vi "transport char run.vi"() -> ()   [LabVIEW 2009]
uses:
  <vilib>/Utility/file.llb/Write To Spreadsheet File (DBL).vi
panel:
  in  "MAXIMUM":ext format="%.2e"
  in  "MINIMUM":ext=-1e-05 format="%_2e"
  out "graphic display 2":cluster{"trace":dbl[], "trace":dbl[]}(graph)
  in  "Y1 axis":string="Id"
  in  "Y2 axis settings":T1={"Y2 axis on/off"=FALSE, "MINIMUM"=-1e-07, "MAXIMUM"=1e-07, "Variable name"="", "LIN or LOG axis"=""} {"MAXIMUM" format="%.2e"; "MINIMUM" format="%.2e"}
  in  "VISA session":refnum<visa-resource-name>="GPIB0::17::INSTR"
  out "graphic display":cluster{"trace":dbl[], "trace":dbl[]}(graph)
  in  "Var2 step settings":T2={"compliance (A)"=0.001, "compliance (V)"=100.0, "start"=0.0, "total points"=7, "step"=-10.0} {"step" format="%.2f"; "start" format="%.2f"; "compliance (V)" format="%.2f"; "compliance (A)" format="%^.2e"}
  in  "wait time parameter":dbl=1.0
  in  "integration time":u32(slide) scale=0.0..2.0
  in  "Var1 sweep settings":T3={"start"=0.0, "stop"=-60.0, "step (linear only)"=-1.0, "sweep spacing (linear: 0)"=0, "sweep mode"=FALSE, "compliance (V)"=100.0, "compliance (A)"=0.001} {"compliance (A)" format="%^.2e"; "compliance (V)" format="%.2f"; "sweep spacing (linear: 0)" items=["linear", "log 10", "log 25", "log 50"]; "step (linear only)" format="%.2f"; "stop" format="%.2f"; "start" format="%.2f"}
  in  "Value (Either V or A) 4":dbl
  in  "Value (Either V or A) 3":dbl
  in  "Value (Either V or A) 2":dbl
  in  "Value (V or A)":dbl
  in  "compliance (A)":dbl=0.001 format="%^.2e"
  in  "compliance (V)":dbl=100.0 format="%^.2e"
  out "error?":errorcluster
  in  "Iname":string="Is"
  in  "Vname":string="Vs"
  in  "Function":u16(ring)=4 items=["disabled", "Var1", "Var2", "Var1'", "Constant"]
  in  "Mode":u16(ring)=4 items=["V", "I", "VPulse", "IPulse", "Common"]
  in  "Iname 4":string="I4"
  in  "Vname 4":string="V4"
  in  "Function 4":u16(ring)=4 items=["disabled", "Var1", "Var2", "Var1'", "Constant"]
  in  "Mode 4":u16(ring) items=["V", "I", "VPulse", "IPulse", "Common"]
  in  "Iname 3":string="Ig"
  in  "Vname 3":string="Vg"
  in  "Function 3":u16(ring)=2 items=["disabled", "Var1", "Var2", "Var1'", "Constant"]
  in  "Mode 3":u16(ring) items=["V", "I", "VPulse", "IPulse", "Common"]
  in  "Iname 2":string="Id"
  in  "Vname 2":string="Vd"
  in  "Function 2":u16(ring)=1 items=["disabled", "Var1", "Var2", "Var1'", "Constant"]
  in  "Mode 2":u16(ring) items=["V", "I", "VPulse", "IPulse", "Common"]
  in  "reset":bool=TRUE
  # "SMU1"
  # "SMU2"
  # "SMU3"
  # "SMU4"
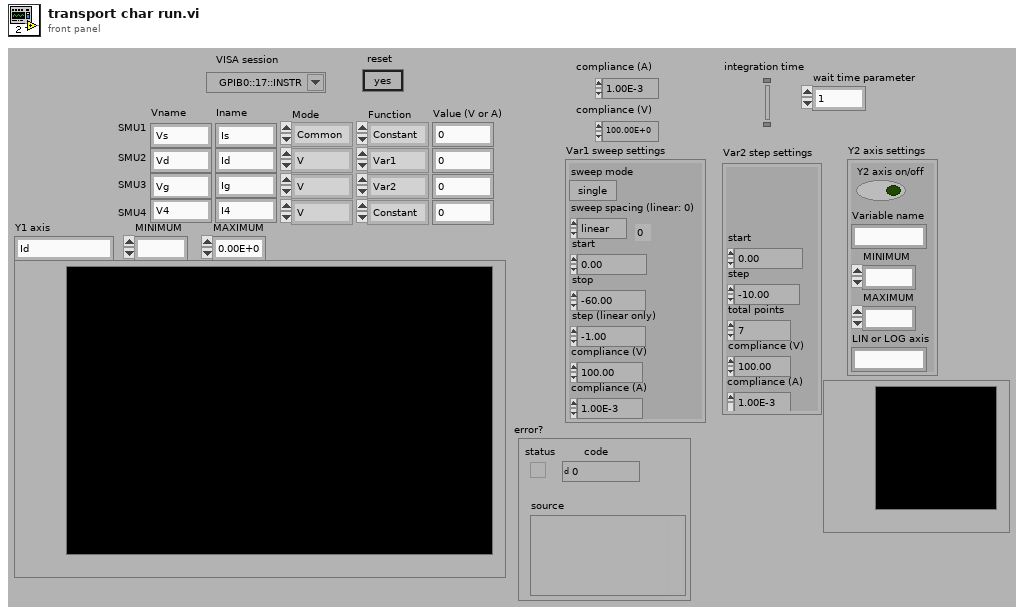
[diagram p1: front panel]
types:
  T1 = cluster{"Y2 axis on/off":bool, "MINIMUM":ext, "MAXIMUM":ext, "Variable name":string, "LIN or LOG axis":string}
  T2 = cluster{"compliance (A)":dbl, "compliance (V)":dbl, "start":dbl, "total points":u16, "step":dbl}
  T3 = cluster{"start":dbl, "stop":dbl, "step (linear only)":dbl, "sweep spacing (linear: 0)":u16, "sweep mode":bool, "compliance (V)":dbl, "compliance (A)":dbl}
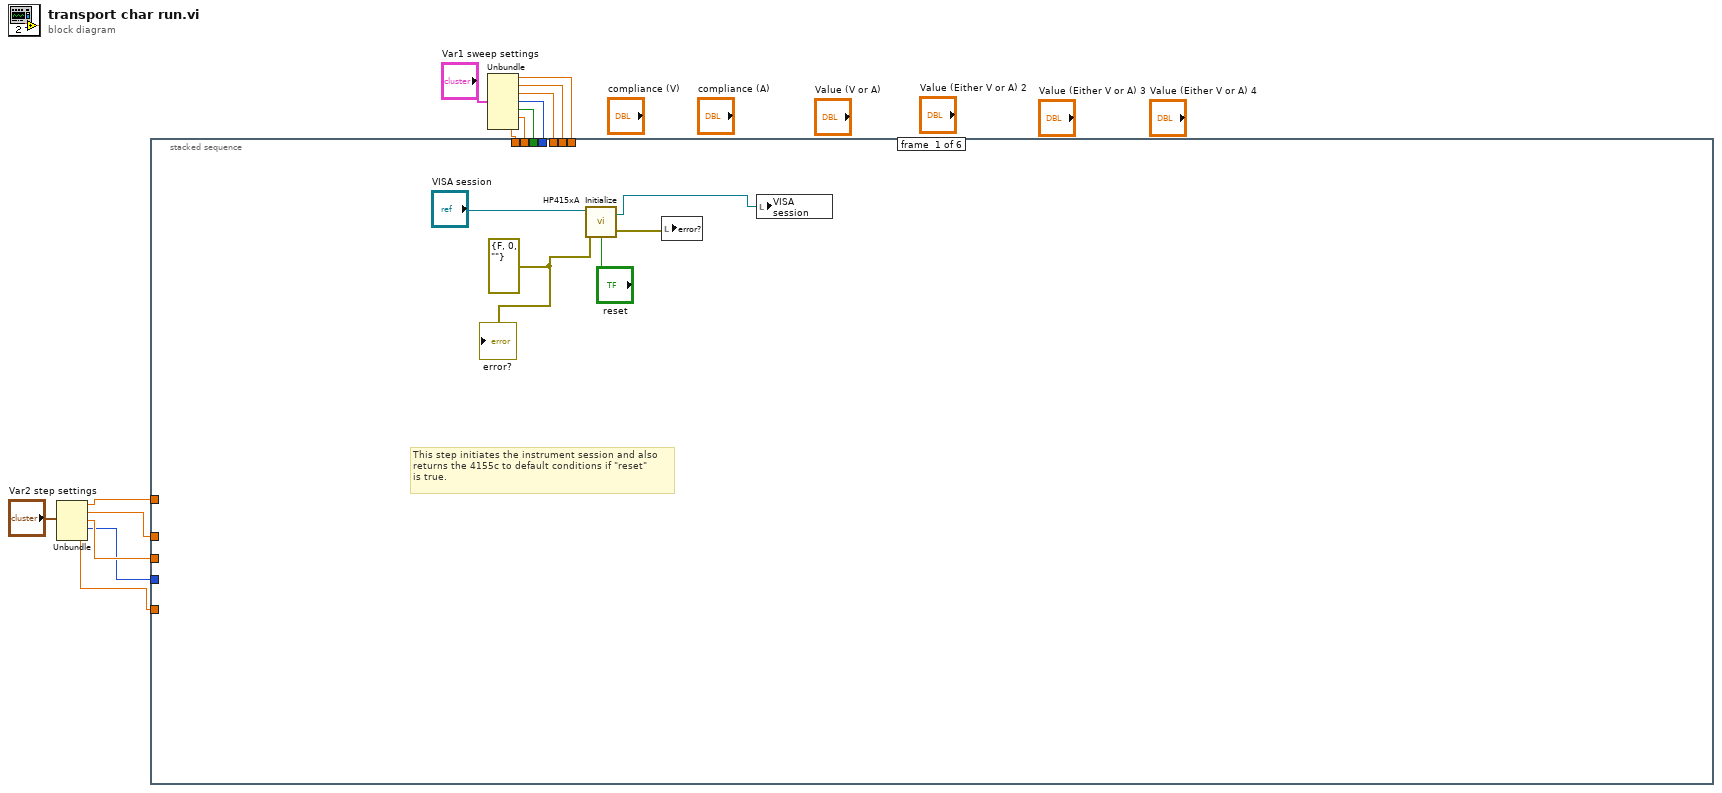
[diagram p0: block diagram]
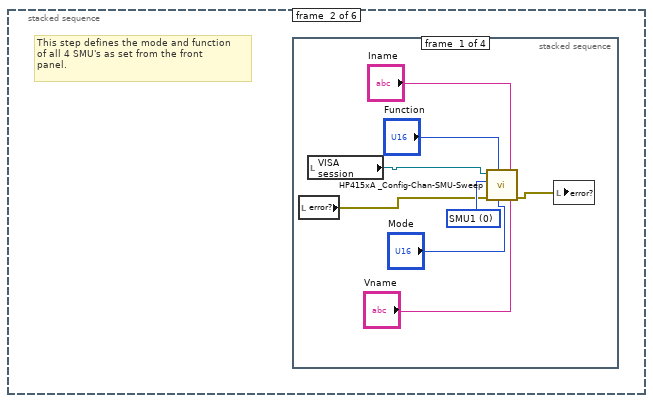
[diagram p2: hidden frame]
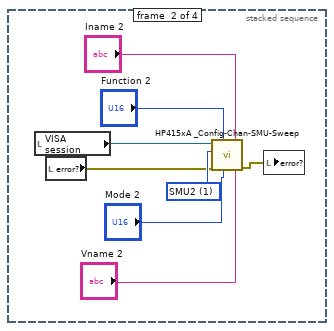
[diagram p3: hidden frame]
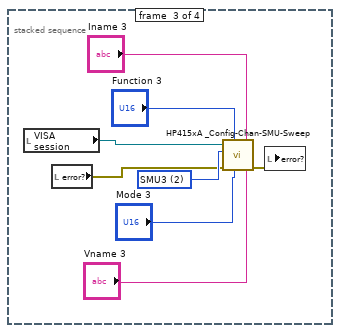
[diagram p4: hidden frame]
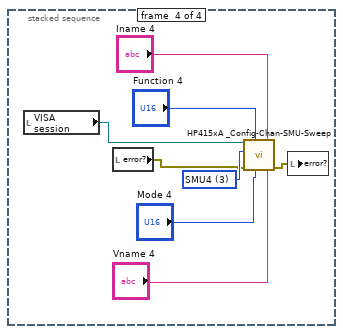
[diagram p5: hidden frame]
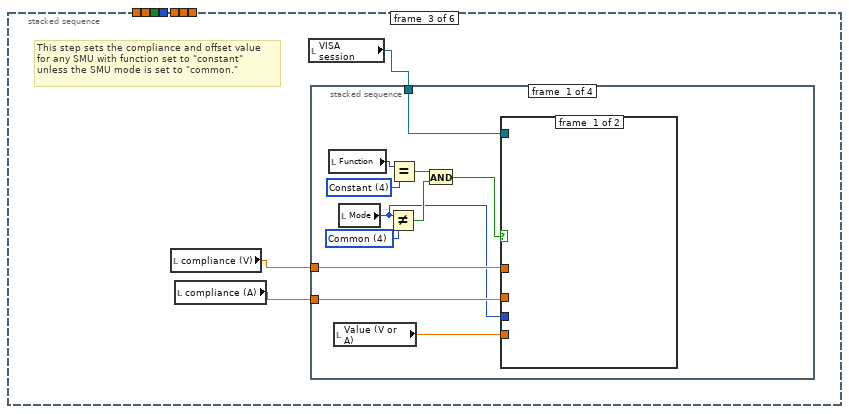
[diagram p6: hidden frame]
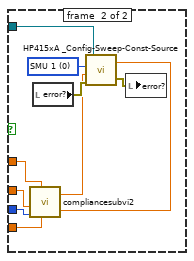
[diagram p7: hidden frame]
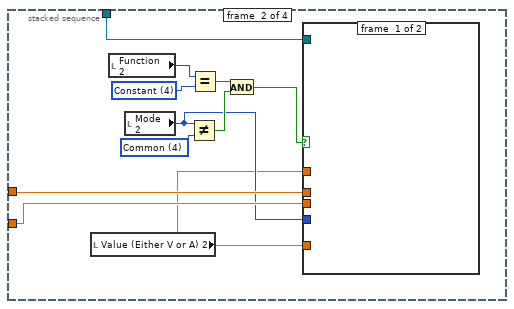
[diagram p8: hidden frame]
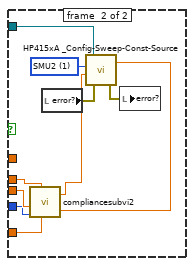
[diagram p9: hidden frame]
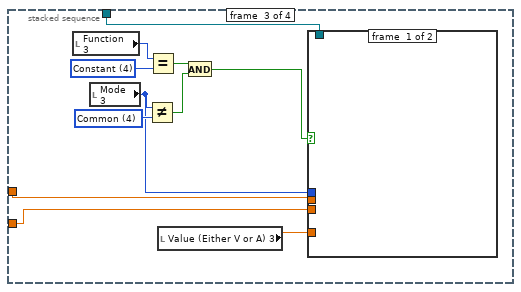
[diagram p10: hidden frame]
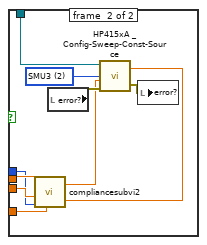
[diagram p11: hidden frame]
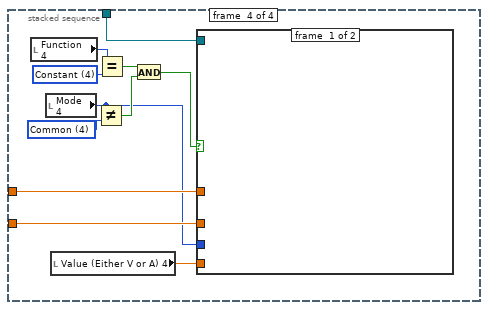
[diagram p12: hidden frame]
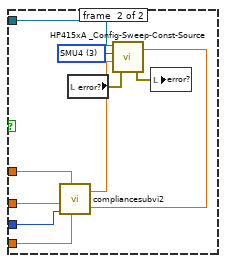
[diagram p13: hidden frame]
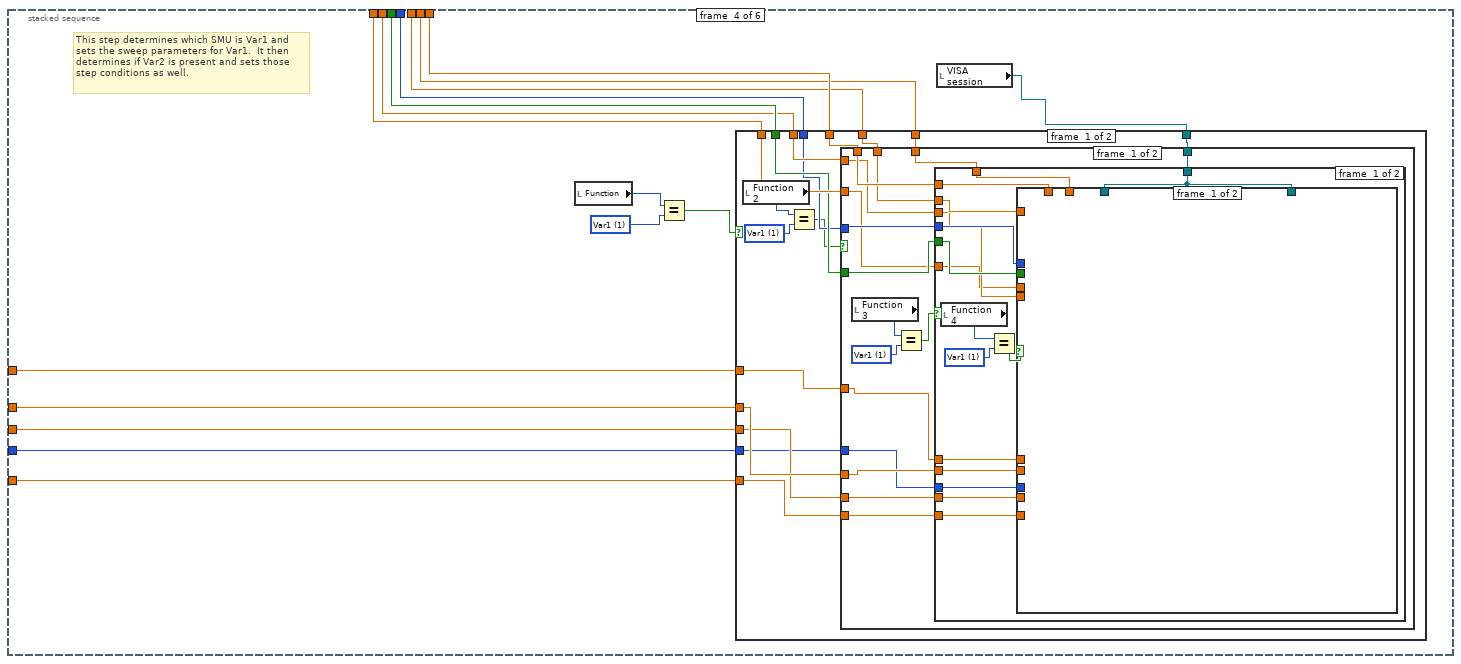
[diagram p14: hidden frame]
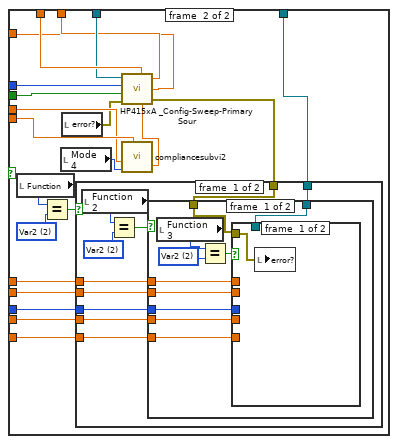
[diagram p15: hidden frame]
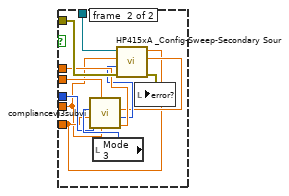
[diagram p16: hidden frame]
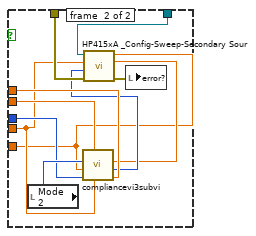
[diagram p17: hidden frame]
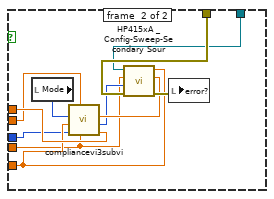
[diagram p18: hidden frame]
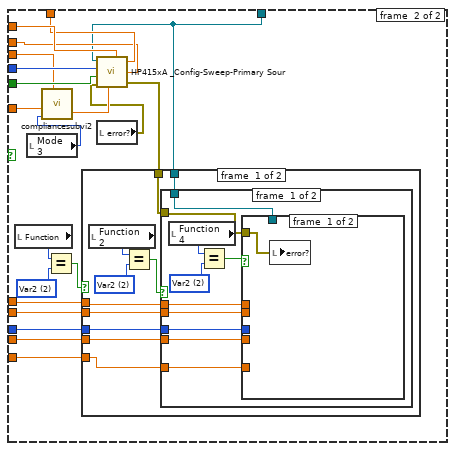
[diagram p19: hidden frame]
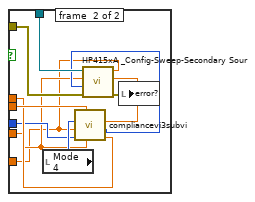
[diagram p20: hidden frame]
diagram:
  n1 = Unbundle("Var2 step settings") -> ("compliance (A)"=w5:dbl, "compliance (V)"=w4:dbl, "start"=w3:dbl, "total points"=w2:u16, "step"=w1:dbl)
  n2 = Unbundle("Var1 sweep settings") -> ("start"=w13:dbl, "stop"=w12:dbl, "step (linear only)"=w11:dbl, "sweep spacing (linear: 0)"=w10:u16, "sweep mode"=w9:bool, "compliance (V)"=w8:dbl, "compliance (A)"=w7:dbl)
  n3 = stacked-sequence {
    tunnel: w13 -> [_ _ _ w150 _ _]
    tunnel: w12 -> [_ _ _ w149 _ _]
    tunnel: w11 -> [_ _ _ w148 _ _]
    tunnel: w10 -> [_ _ _ w147 _ _]
    tunnel: w9 -> [_ _ _ w146 _ _]
    tunnel: w8 -> [_ _ _ w145 _ _]
    tunnel: w7 -> [_ _ _ w144 _ _]
    tunnel: w5 -> [_ _ _ w143 _ _]
    tunnel: w4 -> [_ _ _ w142 _ _]
    tunnel: w3 -> [_ _ _ w141 _ _]
    tunnel: w2 -> [_ _ _ w140 _ _]
    tunnel: w1 -> [_ _ _ w139 _ _]
    frame #0 {
      w18 = errorcluster {"status"=FALSE, "code"=0, "source"=""} ("error out")
      # "This step initiates the instrument session and also\nreturns the 4155c to default conditions if \"reset\"\nis true."
      n4 = call "HP415xA  Initialize.vi"("instrument descriptor"="VISA session", "reset"="reset", "error in (no error)"=w18) -> ("VISA session"=w15:refnum<visa-resource-name>, "error out"=w17:errorcluster)  [unwired: 2 in]
      n5 = local write "error?"(w17) -> ()
      n6 = local write "VISA session"(w15) -> ()
      "error?" <- w18
    }
    frame #1 {
      # "This step defines the mode and function\nof all 4 SMU's as set from the front\npanel."
      n7 = stacked-sequence {
        frame #0 {
          w27 = u32 0 items=["SMU1  ", "SMU2  ", "SMU3  ", "SMU4  ", "SMU5  ", "SMU6  "] ("unit to configure")
          n8 = local read "error?"() -> (w22:errorcluster)
          n9 = local read "VISA session"() -> (w20:refnum<visa-resource-name>)
          n10 = call "HP415xA _Config-Chan-SMU-Sweep.vi"("V name (max 6 chars)"="Vname", "I name (max 6 chars)"="Iname", "mode"="Mode", "function"="Function", "error in (no error)"=w22, "unit to configure"=w27, "VISA session"=w20) -> ("error out"=w21:errorcluster)  [unwired: 2 in]
          n11 = local write "error?"(w21) -> ()
        }
        frame #1 {
          w31 = u32 1 items=["SMU1  ", "SMU2  ", "SMU3  ", "SMU4  ", "SMU5  ", "SMU6  "] ("unit to configure")
          n12 = local read "VISA session"() -> (w28:refnum<visa-resource-name>)
          n13 = local read "error?"() -> (w29:errorcluster)
          n14 = call "HP415xA _Config-Chan-SMU-Sweep.vi"("V name (max 6 chars)"="Vname 2", "I name (max 6 chars)"="Iname 2", "mode"="Mode 2", "function"="Function 2", "error in (no error)"=w29, "unit to configure"=w31, "VISA session"=w28) -> ("error out"=w30:errorcluster)  [unwired: 2 in]
          n15 = local write "error?"(w30) -> ()
        }
        frame #2 {
          w39 = u32 2 items=["SMU1  ", "SMU2  ", "SMU3  ", "SMU4  ", "SMU5  ", "SMU6  "] ("unit to configure")
          n16 = local read "VISA session"() -> (w36:refnum<visa-resource-name>)
          n17 = local read "error?"() -> (w37:errorcluster)
          n18 = call "HP415xA _Config-Chan-SMU-Sweep.vi"("V name (max 6 chars)"="Vname 3", "I name (max 6 chars)"="Iname 3", "mode"="Mode 3", "function"="Function 3", "error in (no error)"=w37, "unit to configure"=w39, "VISA session"=w36) -> ("error out"=w38:errorcluster)  [unwired: 2 in]
          n19 = local write "error?"(w38) -> ()
        }
        frame #3 {
          w47 = u32 3 items=["SMU1  ", "SMU2  ", "SMU3  ", "SMU4  ", "SMU5  ", "SMU6  "] ("unit to configure")
          n20 = local read "VISA session"() -> (w44:refnum<visa-resource-name>)
          n21 = local read "error?"() -> (w46:errorcluster)
          n22 = call "HP415xA _Config-Chan-SMU-Sweep.vi"("V name (max 6 chars)"="Vname 4", "I name (max 6 chars)"="Iname 4", "mode"="Mode 4", "function"="Function 4", "error in (no error)"=w46, "unit to configure"=w47, "VISA session"=w44) -> ("error out"=w45:errorcluster)  [unwired: 2 in]
          n23 = local write "error?"(w45) -> ()
        }
      }
    }
    frame #2 {
      # "This step sets the compliance and offset value\nfor any SMU with function set to \"constant\"\nunless the SMU mode is set to \"common.\""
      n24 = local read "compliance (V)"() -> (w53:dbl)
      n25 = local read "compliance (A)"() -> (w54:dbl)
      n26 = local read "VISA session"() -> (w52:refnum<visa-resource-name>)
      n27 = stacked-sequence {
        tunnel: w52 -> [w63 w83 w102 w122]
        tunnel: w54 -> [w57 w79 w100 w120]
        tunnel: w53 -> [w56 w78 w99 w121]
        frame #0 {
          w61 = u16 4 items=["V", "I", "VPulse", "IPulse", "Common"] ("Mode")
          w65 = u16 4 items=["disabled", "Var1", "Var2", "Var1'", "Constant"] ("Function")
          n28 = local read "Function"() -> (w64:u16)
          n29 = local read "Value (V or A)"() -> (w58:dbl)
          n30 = local read "Mode"() -> (w55:u16)
          n31 = Not Equal?(x=w55, y=w61) -> (x != y?=w60:bool)
          n32 = Equal?(x=w64, y=w65) -> (x = y?=w62:bool)
          n33 = And(x=w62, y=w60) -> (x .and. y?=w59:bool)
          n34 = case shown="False" w59 {
            tunnel: w63 -> [_ w75]
            tunnel: w56 -> [_ w71]
            tunnel: w57 -> [_ w70]
            tunnel: w58 -> [_ w67]
            tunnel: w55 -> [_ w68]
            frame #0 {
            }
            frame #1 {
              w74 = u16 0 items=["SMU 1", "SMU2", "SMU3", "SMU4", "SMU5", "SMU6", "VSU1", "VSU2"] ("unit (SMU1:0)")
              n35 = call "compliancesubvi2.vi"("Value1"=w67, "compliance (V)"=w71, "Mode"=w68, "compliance (A)"=w70) -> ("compliance"=w69:dbl, "constant"=w66:dbl)  [unwired: 2 in]
              n36 = local read "error?"() -> (w73:errorcluster)
              n37 = call "HP415xA _Config-Sweep-Const-Source.vi"("compliance (SMUs only)"=w69, "error in (no error)"=w73, "source (V or A)"=w66, "unit (SMU1:0)"=w74, "VISA session"=w75) -> ("error out"=w72:errorcluster)
              n38 = local write "error?"(w72) -> ()
            }
          }
        }
        frame #1 {
          w80 = u16 4 items=["V", "I", "VPulse", "IPulse", "Common"] ("Mode 2")
          w81 = u16 4 items=["disabled", "Var1", "Var2", "Var1'", "Constant"] ("Function 2")
          n39 = local read "Value (Either V or A) 2"() -> (w76:dbl)
          n40 = local read "Function 2"() -> (w82:u16)
          n41 = local read "Mode 2"() -> (w77:u16)
          n42 = Not Equal?(x=w77, y=w80) -> (x != y?=w85:bool)
          n43 = Equal?(x=w82, y=w81) -> (x = y?=w86:bool)
          n44 = And(x=w86, y=w85) -> (x .and. y?=w84:bool)
          n45 = case shown="False" w84 {
            tunnel: w83 -> [_ w96]
            tunnel: w78 -> [_ w94]
            tunnel: w79 -> [_ w93]
            tunnel: w76 -> [_ _]
            tunnel: w77 -> [_ w89]
            tunnel: w76 -> [_ w88]
            frame #0 {
            }
            frame #1 {
              w95 = u16 1 items=["SMU 1", "SMU2", "SMU3", "SMU4", "SMU5", "SMU6", "VSU1", "VSU2"] ("unit (SMU1:0)")
              n46 = call "compliancesubvi2.vi"("Value1"=w88, "compliance (V)"=w94, "Mode"=w89, "compliance (A)"=w93) -> ("compliance"=w92:dbl, "constant"=w87:dbl)  [unwired: 2 in]
              n47 = local read "error?"() -> (w91:errorcluster)
              n48 = call "HP415xA _Config-Sweep-Const-Source.vi"("compliance (SMUs only)"=w92, "error in (no error)"=w91, "source (V or A)"=w87, "unit (SMU1:0)"=w95, "VISA session"=w96) -> ("error out"=w90:errorcluster)
              n49 = local write "error?"(w90) -> ()
            }
          }
        }
        frame #2 {
          w104 = u16 4 items=["V", "I", "VPulse", "IPulse", "Common"] ("Mode 2")
          w105 = u16 4 items=["disabled", "Var1", "Var2", "Var1'", "Constant"] ("Function 2")
          n50 = local read "Function 3"() -> (w103:u16)
          n51 = local read "Mode 3"() -> (w98:u16)
          n52 = Not Equal?(x=w98, y=w104) -> (x != y?=w106:bool)
          n53 = Equal?(x=w103, y=w105) -> (x = y?=w107:bool)
          n54 = local read "Value (Either V or A) 3"() -> (w101:dbl)
          n55 = And(x=w107, y=w106) -> (x .and. y?=w97:bool)
          n56 = case shown="False" w97 {
            tunnel: w102 -> [_ w115]
            tunnel: w101 -> [_ w109]
            tunnel: w100 -> [_ w112]
            tunnel: w99 -> [_ w111]
            tunnel: w98 -> [_ w110]
            frame #0 {
            }
            frame #1 {
              w114 = u16 2 items=["SMU 1", "SMU2", "SMU3", "SMU4", "SMU5", "SMU6", "VSU1", "VSU2"] ("unit (SMU1:0)")
              n57 = call "compliancesubvi2.vi"("Value1"=w109, "compliance (V)"=w111, "Mode"=w110, "compliance (A)"=w112) -> ("compliance"=w113:dbl, "constant"=w108:dbl)  [unwired: 2 in]
              n58 = local read "error?"() -> (w117:errorcluster)
              n59 = call "HP415xA _Config-Sweep-Const-Source.vi"("compliance (SMUs only)"=w113, "error in (no error)"=w117, "source (V or A)"=w108, "unit (SMU1:0)"=w114, "VISA session"=w115) -> ("error out"=w116:errorcluster)
              n60 = local write "error?"(w116) -> ()
            }
          }
        }
        frame #3 {
          w124 = u16 4 items=["V", "I", "VPulse", "IPulse", "Common"] ("Mode 4")
          w125 = u16 4 items=["disabled", "Var1", "Var2", "Var1'", "Constant"] ("Function 4")
          n61 = local read "Function 4"() -> (w126:u16)
          n62 = local read "Mode 4"() -> (w119:u16)
          n63 = local read "Value (Either V or A) 4"() -> (w118:dbl)
          n64 = Not Equal?(x=w119, y=w124) -> (x != y?=w127:bool)
          n65 = Equal?(x=w126, y=w125) -> (x = y?=w128:bool)
          n66 = And(x=w128, y=w127) -> (x .and. y?=w123:bool)
          n67 = case shown="True" w123 {
            tunnel: w122 -> [_ w137]
            tunnel: w121 -> [_ w133]
            tunnel: w120 -> [_ w134]
            tunnel: w119 -> [_ w132]
            tunnel: w118 -> [_ w131]
            frame #0 {
            }
            frame #1 {
              w138 = u16 3 items=["SMU 1", "SMU2", "SMU3", "SMU4", "SMU5", "SMU6", "VSU1", "VSU2"] ("unit (SMU1:0)")
              n68 = call "compliancesubvi2.vi"("Value1"=w131, "compliance (V)"=w133, "Mode"=w132, "compliance (A)"=w134) -> ("compliance"=w130:dbl, "constant"=w129:dbl)  [unwired: 2 in]
              n69 = local read "error?"() -> (w136:errorcluster)
              n70 = call "HP415xA _Config-Sweep-Const-Source.vi"("compliance (SMUs only)"=w130, "error in (no error)"=w136, "source (V or A)"=w129, "unit (SMU1:0)"=w138, "VISA session"=w137) -> ("error out"=w135:errorcluster)
              n71 = local write "error?"(w135) -> ()
            }
          }
        }
      }
    }
    frame #3 {
      w154 = u16 1 items=["disabled", "Var1", "Var2", "Var1'", "Constant"] ("Function")
      # "This step determines which SMU is Var1 and\nsets the sweep parameters for Var1.  It then\ndetermines if Var2 is present and sets those\nstep conditions as well."
      n72 = local read "Function"() -> (w153:u16)
      n73 = Equal?(x=w153, y=w154) -> (x = y?=w152:bool)
      n74 = local read "VISA session"() -> (w151:refnum<visa-resource-name>)
      n75 = case shown="False" w152 {
        tunnel: w145 -> [w167 w443]
        tunnel: w144 -> [w168 w442]
        tunnel: w147 -> [w165 w441]
        tunnel: w146 -> [w166 w440]
        tunnel: w148 -> [w162 w439]
        tunnel: w149 -> [w161 w438]
        tunnel: w150 -> [w163 w437]
        tunnel: w151 -> [w164 w426]
        tunnel: w143 -> [w159 w432]
        tunnel: w142 -> [w158 w431]
        tunnel: w141 -> [w157 w430]
        tunnel: w140 -> [w156 w429]
        tunnel: w139 -> [w155 w428]
        frame #0 {
          w170 = u16 1 items=["disabled", "Var1", "Var2", "Var1'", "Constant"] ("Function")
          n76 = local read "Function 2"() -> (w169:u16)
          n77 = Equal?(x=w169, y=w170) -> (x = y?=w160:bool)
          n78 = case shown="False" w160 {
            tunnel: w168 -> [w176 w369]
            tunnel: w167 -> [w177 w368]
            tunnel: w166 -> [w178 w367]
            tunnel: w165 -> [w179 w366]
            tunnel: w164 -> [w183 w355]
            tunnel: w163 -> [w182 w365]
            tunnel: w162 -> [w180 w364]
            tunnel: w161 -> [w181 w363]
            tunnel: w159 -> [w175 w358]
            tunnel: w158 -> [w174 w357]
            tunnel: w157 -> [w172 w356]
            tunnel: w156 -> [w173 w353]
            tunnel: w155 -> [w171 w352]
            frame #0 {
              w186 = u16 1 items=["disabled", "Var1", "Var2", "Var1'", "Constant"] ("Function")
              n79 = local read "Function 3"() -> (w185:u16)
              n80 = Equal?(x=w185, y=w186) -> (x = y?=w184:bool)
              n81 = case shown="True" w184 {
                tunnel: w183 -> [w187 w280]
                tunnel: w182 -> [w199 w297]
                tunnel: w181 -> [w196 w296]
                tunnel: w180 -> [w195 w295]
                tunnel: w179 -> [w198 w294]
                tunnel: w178 -> [w197 w293]
                tunnel: w177 -> [w194 w292]
                tunnel: w176 -> [w193 w291]
                tunnel: w175 -> [w192 w284]
                tunnel: w174 -> [w191 w283]
                tunnel: w173 -> [w190 w282]
                tunnel: w172 -> [w189 w279]
                tunnel: w171 -> [w188 w278]
                frame #0 {
                  w202 = u16 1 items=["disabled", "Var1", "Var2", "Var1'", "Constant"] ("Function")
                  n82 = local read "Function 4"() -> (w201:u16)
                  n83 = Equal?(x=w201, y=w202) -> (x = y?=w200:bool)
                  n84 = case shown="True" w200 {
                    tunnel: w199 -> [_ w221]
                    tunnel: w187 -> [_ w220]
                    tunnel: w198 -> [_ w219]
                    tunnel: w197 -> [_ w218]
                    tunnel: w196 -> [_ w217]
                    tunnel: w195 -> [_ w216]
                    tunnel: w194 -> [_ w215]
                    tunnel: w193 -> [_ w214]
                    tunnel: w192 -> [_ w209]
                    tunnel: w191 -> [_ w208]
                    tunnel: w190 -> [_ w207]
                    tunnel: w189 -> [_ w206]
                    tunnel: w188 -> [_ w205]
                    tunnel: w187 -> [_ w203]
                    frame #0 {
                    }
                    frame #1 {
                      w212 = u16 2 items=["disabled", "Var1", "Var2", "Var1'", "Constant"] ("Function")
                      n85 = local read "Function"() -> (w211:u16)
                      n86 = Equal?(x=w211, y=w212) -> (x = y?=w210:bool)
                      n87 = local read "Mode 4"() -> (w223:u16)
                      n88 = local read "error?"() -> (w213:errorcluster)
                      n89 = call "compliancesubvi2.vi"("compliance (V)"=w215, "Mode"=w223, "compliance (A)"=w214) -> ("compliance"=w222:dbl)  [unwired: 3 in, 1 out]
                      n90 = call "HP415xA _Config-Sweep-Primary Sour.vi"("step (linear only)"=w216, "stop"=w217, "start"=w221, "compliance"=w222, "error in (no error)"=w213, "sweep mode"=w218, "sweep spacing (linear: 0)"=w219, "VISA session"=w220) -> ("error out"=w204:errorcluster)  [unwired: 2 in]
                      n91 = case shown="False" w210 {
                        tunnel: w209 -> [w230 w273]
                        tunnel: w208 -> [w229 w268]
                        tunnel: w207 -> [w228 w267]
                        tunnel: w206 -> [w227 w269]
                        tunnel: w205 -> [w226 w272]
                        tunnel: w204 -> [w225 w275]
                        tunnel: w203 -> [w224 w274]
                        frame #0 {
                          w233 = u16 2 items=["disabled", "Var1", "Var2", "Var1'", "Constant"] ("Function")
                          n92 = local read "Function 2"() -> (w232:u16)
                          n93 = Equal?(x=w232, y=w233) -> (x = y?=w231:bool)
                          n94 = case shown="False" w231 {
                            tunnel: w230 -> [w241 w261]
                            tunnel: w229 -> [w240 w262]
                            tunnel: w228 -> [w239 w260]
                            tunnel: w227 -> [w238 w258]
                            tunnel: w226 -> [w237 w256]
                            tunnel: w225 -> [w236 w266]
                            tunnel: w224 -> [w234 w265]
                            frame #0 {
                              w243 = u16 2 items=["disabled", "Var1", "Var2", "Var1'", "Constant"] ("Function")
                              n95 = local read "Function 3"() -> (w235:u16)
                              n96 = Equal?(x=w235, y=w243) -> (x = y?=w242:bool)
                              n97 = case shown="True" w242 {
                                tunnel: w241 -> [_ w249]
                                tunnel: w240 -> [_ w250]
                                tunnel: w239 -> [_ w251]
                                tunnel: w238 -> [_ w245]
                                tunnel: w237 -> [_ w246]
                                tunnel: w236 -> [w244 w255]
                                tunnel: w234 -> [_ w254]
                                frame #0 {
                                n98 = local write "error?"(w244) -> ()
                                }
                                frame #1 {
                                n99 = local read "Mode 3"() -> (w253:u16)
                                n100 = call "compliancevi3subvi.vi"("compliance (A)"=w249, "start"=w245, "compliance (V)"=w250, "total points"=w251, "step"=w246, "Mode"=w253) -> ("total points 2"=w248:u16, "compliance"=w247:dbl)  [unwired: 1 in, 1 out]
                                n101 = call "HP415xA _Config-Sweep-Secondary Sour.vi"("compliance"=w247, "step"=w246, "error in (no error)"=w255, "total points"=w248, "start"=w245, "VISA session"=w254) -> ("error out"=w252:errorcluster)  [unwired: 1 in]
                                n102 = local write "error?"(w252) -> ()
                                }
                              }
                            }
                            frame #1 {
                              n103 = local read "Mode 2"() -> (w264:u16)
                              n104 = call "compliancevi3subvi.vi"("compliance (A)"=w261, "start"=w258, "compliance (V)"=w262, "total points"=w260, "step"=w256, "Mode"=w264) -> ("total points 2"=w259:u16, "compliance"=w257:dbl)  [unwired: 1 in, 1 out]
                              n105 = call "HP415xA _Config-Sweep-Secondary Sour.vi"("compliance"=w257, "step"=w256, "error in (no error)"=w266, "total points"=w259, "start"=w258, "VISA session"=w265) -> ("error out"=w263:errorcluster)  [unwired: 1 in]
                              n106 = local write "error?"(w263) -> ()
                            }
                          }
                        }
                        frame #1 {
                          n107 = local read "Mode"() -> (w277:u16)
                          n108 = call "compliancevi3subvi.vi"("compliance (A)"=w273, "start"=w269, "compliance (V)"=w268, "total points"=w267, "step"=w272, "Mode"=w277) -> ("total points 2"=w270:u16, "compliance"=w271:dbl)  [unwired: 1 in, 1 out]
                          n109 = call "HP415xA _Config-Sweep-Secondary Sour.vi"("compliance"=w271, "step"=w272, "error in (no error)"=w275, "total points"=w270, "start"=w269, "VISA session"=w274) -> ("error out"=w276:errorcluster)  [unwired: 1 in]
                          n110 = local write "error?"(w276) -> ()
                        }
                      }
                    }
                  }
                }
                frame #1 {
                  w287 = u16 2 items=["disabled", "Var1", "Var2", "Var1'", "Constant"] ("Function")
                  n111 = local read "Function"() -> (w286:u16)
                  n112 = local read "Mode 3"() -> (w289:u16)
                  n113 = call "compliancesubvi2.vi"("compliance (V)"=w292, "Mode"=w289, "compliance (A)"=w291) -> ("compliance"=w290:dbl)  [unwired: 3 in, 1 out]
                  n114 = Equal?(x=w286, y=w287) -> (x = y?=w285:bool)
                  n115 = local read "error?"() -> (w288:errorcluster)
                  n116 = call "HP415xA _Config-Sweep-Primary Sour.vi"("step (linear only)"=w295, "stop"=w296, "start"=w297, "compliance"=w290, "error in (no error)"=w288, "sweep mode"=w293, "sweep spacing (linear: 0)"=w294, "VISA session"=w280) -> ("error out"=w281:errorcluster)  [unwired: 2 in]
                  n117 = case shown="False" w285 {
                    tunnel: w284 -> [w302 w347]
                    tunnel: w283 -> [w301 w346]
                    tunnel: w282 -> [w299 w345]
                    tunnel: w281 -> [w304 w350]
                    tunnel: w280 -> [w303 w349]
                    tunnel: w279 -> [w298 w342]
                    tunnel: w278 -> [w300 w341]
                    frame #0 {
                      w307 = u16 2 items=["disabled", "Var1", "Var2", "Var1'", "Constant"] ("Function")
                      n118 = local read "Function 2"() -> (w306:u16)
                      n119 = Equal?(x=w306, y=w307) -> (x = y?=w305:bool)
                      n120 = case shown="True" w305 {
                        tunnel: w304 -> [w314 w339]
                        tunnel: w303 -> [w313 w338]
                        tunnel: w302 -> [w312 w334]
                        tunnel: w301 -> [w311 w335]
                        tunnel: w300 -> [w308 w333]
                        tunnel: w299 -> [w310 w336]
                        tunnel: w298 -> [w309 w332]
                        frame #0 {
                          w317 = u16 2 items=["disabled", "Var1", "Var2", "Var1'", "Constant"] ("Function")
                          n121 = local read "Function 4"() -> (w316:u16)
                          n122 = Equal?(x=w316, y=w317) -> (x = y?=w315:bool)
                          n123 = case shown="True" w315 {
                            tunnel: w314 -> [w318 w327]
                            tunnel: w313 -> [_ w328]
                            tunnel: w312 -> [_ w324]
                            tunnel: w311 -> [_ w325]
                            tunnel: w310 -> [_ w323]
                            tunnel: w309 -> [_ w320]
                            tunnel: w308 -> [_ w319]
                            frame #0 {
                              n124 = local write "error?"(w318) -> ()
                            }
                            frame #1 {
                              n125 = local read "Mode 4"() -> (w329:u16)
                              n126 = call "compliancevi3subvi.vi"("compliance (A)"=w324, "start"=w320, "compliance (V)"=w325, "total points"=w323, "step"=w319, "Mode"=w329) -> ("total points 2"=w322:u16, "compliance"=w321:dbl)  [unwired: 1 in, 1 out]
                              n127 = call "HP415xA _Config-Sweep-Secondary Sour.vi"("compliance"=w321, "step"=w319, "error in (no error)"=w327, "total points"=w322, "start"=w320, "VISA session"=w328) -> ("error out"=w326:errorcluster)  [unwired: 1 in]
                              n128 = local write "error?"(w326) -> ()
                            }
                          }
                        }
                        frame #1 {
                          n129 = local read "Mode 2"() -> (w340:u16)
                          n130 = call "compliancevi3subvi.vi"("compliance (A)"=w334, "start"=w332, "compliance (V)"=w335, "total points"=w336, "step"=w333, "Mode"=w340) -> ("total points 2"=w331:u16, "compliance"=w330:dbl)  [unwired: 1 in, 1 out]
                          n131 = call "HP415xA _Config-Sweep-Secondary Sour.vi"("compliance"=w330, "step"=w333, "error in (no error)"=w339, "total points"=w331, "start"=w332, "VISA session"=w338) -> ("error out"=w337:errorcluster)  [unwired: 1 in]
                          n132 = local write "error?"(w337) -> ()
                        }
                      }
                    }
                    frame #1 {
                      n133 = local read "Mode"() -> (w351:u16)
                      n134 = call "compliancevi3subvi.vi"("compliance (A)"=w347, "start"=w342, "compliance (V)"=w346, "total points"=w345, "step"=w341, "Mode"=w351) -> ("total points 2"=w344:u16, "compliance"=w343:dbl)  [unwired: 1 in, 1 out]
                      n135 = call "HP415xA _Config-Sweep-Secondary Sour.vi"("compliance"=w343, "step"=w341, "error in (no error)"=w350, "total points"=w344, "start"=w342, "VISA session"=w349) -> ("error out"=w348:errorcluster)  [unwired: 1 in]
                      n136 = local write "error?"(w348) -> ()
                    }
                  }
                }
              }
            }
            frame #1 {
              w361 = u16 2 items=["disabled", "Var1", "Var2", "Var1'", "Constant"] ("Function")
              n137 = local read "Mode 2"() -> (w370:u16)
              n138 = local read "Function"() -> (w360:u16)
              n139 = Equal?(x=w360, y=w361) -> (x = y?=w359:bool)
              n140 = local read "error?"() -> (w362:errorcluster)
              n141 = call "compliancesubvi2.vi"("compliance (V)"=w368, "Mode"=w370, "compliance (A)"=w369) -> ("compliance"=w371:dbl)  [unwired: 3 in, 1 out]
              n142 = call "HP415xA _Config-Sweep-Primary Sour.vi"("step (linear only)"=w364, "stop"=w363, "start"=w365, "compliance"=w371, "error in (no error)"=w362, "sweep mode"=w367, "sweep spacing (linear: 0)"=w366, "VISA session"=w355) -> ("error out"=w354:errorcluster)  [unwired: 2 in]
              n143 = case shown="False" w359 {
                tunnel: w358 -> [w377 w420]
                tunnel: w357 -> [w376 w419]
                tunnel: w356 -> [w374 w415]
                tunnel: w355 -> [w379 w425]
                tunnel: w354 -> [w373 w424]
                tunnel: w353 -> [w375 w421]
                tunnel: w352 -> [w372 w417]
                frame #0 {
                  w381 = u16 2 items=["disabled", "Var1", "Var2", "Var1'", "Constant"] ("Function")
                  n144 = local read "Function 3"() -> (w380:u16)
                  n145 = Equal?(x=w380, y=w381) -> (x = y?=w378:bool)
                  n146 = case shown="False" w378 {
                    tunnel: w379 -> [w387 w413]
                    tunnel: w377 -> [w386 w410]
                    tunnel: w376 -> [w384 w408]
                    tunnel: w375 -> [w385 w409]
                    tunnel: w374 -> [w382 w406]
                    tunnel: w373 -> [w388 w412]
                    tunnel: w372 -> [w383 w404]
                    frame #0 {
                      w391 = u16 2 items=["disabled", "Var1", "Var2", "Var1'", "Constant"] ("Function")
                      n147 = local read "Function 4"() -> (w390:u16)
                      n148 = Equal?(x=w390, y=w391) -> (x = y?=w389:bool)
                      n149 = case shown="True" w389 {
                        tunnel: w388 -> [w392 w403]
                        tunnel: w387 -> [_ w402]
                        tunnel: w386 -> [_ w399]
                        tunnel: w385 -> [_ w400]
                        tunnel: w384 -> [_ w398]
                        tunnel: w383 -> [_ w394]
                        tunnel: w382 -> [_ w395]
                        frame #0 {
                          n150 = local write "error?"(w392) -> ()
                        }
                        frame #1 {
                          n151 = local read "Mode 4"() -> (w397:u16)
                          n152 = call "compliancevi3subvi.vi"("compliance (A)"=w399, "start"=w395, "compliance (V)"=w398, "total points"=w400, "step"=w394, "Mode"=w397) -> ("total points 2"=w396:u16, "compliance"=w393:dbl)  [unwired: 1 in, 1 out]
                          n153 = call "HP415xA _Config-Sweep-Secondary Sour.vi"("compliance"=w393, "step"=w394, "error in (no error)"=w403, "total points"=w396, "start"=w395, "VISA session"=w402) -> ("error out"=w401:errorcluster)  [unwired: 1 in]
                          n154 = local write "error?"(w401) -> ()
                        }
                      }
                    }
                    frame #1 {
                      n155 = local read "Mode 3"() -> (w414:u16)
                      n156 = call "compliancevi3subvi.vi"("compliance (A)"=w410, "start"=w406, "compliance (V)"=w408, "total points"=w409, "step"=w404, "Mode"=w414) -> ("total points 2"=w407:u16, "compliance"=w405:dbl)  [unwired: 1 in, 1 out]
                      n157 = call "HP415xA _Config-Sweep-Secondary Sour.vi"("compliance"=w405, "step"=w404, "error in (no error)"=w412, "total points"=w407, "start"=w406, "VISA session"=w413) -> ("error out"=w411:errorcluster)  [unwired: 1 in]
                      n158 = local write "error?"(w411) -> ()
                    }
                  }
                }
                frame #1 {
                  n159 = local read "Mode"() -> (w422:u16)
                  n160 = call "compliancevi3subvi.vi"("compliance (A)"=w420, "start"=w415, "compliance (V)"=w419, "total points"=w421, "step"=w417, "Mode"=w422) -> ("total points 2"=w416:u16, "compliance"=w418:dbl)  [unwired: 1 in, 1 out]
                  n161 = call "HP415xA _Config-Sweep-Secondary Sour.vi"("compliance"=w418, "step"=w417, "error in (no error)"=w424, "total points"=w416, "start"=w415, "VISA session"=w425) -> ("error out"=w423:errorcluster)  [unwired: 1 in]
                  n162 = local write "error?"(w423) -> ()
                }
              }
            }
          }
        }
        frame #1 {
          w434 = u16 2 items=["disabled", "Var1", "Var2", "Var1'", "Constant"] ("Function 2")
          n163 = local read "error?"() -> (w436:errorcluster)
          n164 = local read "Mode"() -> (w444:u16)
          n165 = call "compliancesubvi2.vi"("compliance (V)"=w443, "Mode"=w444, "compliance (A)"=w442) -> ("compliance"=w445:dbl)  [unwired: 3 in, 1 out]
          n166 = local read "Function 2"() -> (w435:u16)
          n167 = call "HP415xA _Config-Sweep-Primary Sour.vi"("step (linear only)"=w439, "stop"=w438, "start"=w437, "compliance"=w445, "error in (no error)"=w436, "sweep mode"=w440, "sweep spacing (linear: 0)"=w441, "VISA session"=w426) -> ("error out"=w427:errorcluster)  [unwired: 2 in]
          n168 = Equal?(x=w435, y=w434) -> (x = y?=w433:bool)
          n169 = case shown="True" w433 {
            tunnel: w432 -> [w451 w495]
            tunnel: w431 -> [w452 w494]
            tunnel: w430 -> [w449 w491]
            tunnel: w429 -> [w450 w493]
            tunnel: w428 -> [w448 w489]
            tunnel: w427 -> [w447 w498]
            tunnel: w426 -> [w446 w496]
            frame #0 {
              w455 = u16 2 items=["disabled", "Var1", "Var2", "Var1'", "Constant"] ("Function 2")
              n170 = local read "Function 3"() -> (w454:u16)
              n171 = Equal?(x=w454, y=w455) -> (x = y?=w453:bool)
              n172 = case shown="True" w453 {
                tunnel: w452 -> [w460 w478]
                tunnel: w451 -> [w461 w479]
                tunnel: w450 -> [w458 w484]
                tunnel: w449 -> [w459 w481]
                tunnel: w448 -> [w457 w480]
                tunnel: w447 -> [w462 w487]
                tunnel: w446 -> [w456 w485]
                frame #0 {
                  w465 = u16 2 items=["disabled", "Var1", "Var2", "Var1'", "Constant"] ("Function 2")
                  n173 = local read "Function 4"() -> (w464:u16)
                  n174 = Equal?(x=w464, y=w465) -> (x = y?=w463:bool)
                  n175 = case shown="False" w463 {
                    tunnel: w462 -> [w466 w477]
                    tunnel: w461 -> [_ w467]
                    tunnel: w460 -> [_ w468]
                    tunnel: w459 -> [_ w469]
                    tunnel: w458 -> [_ w474]
                    tunnel: w457 -> [_ w471]
                    tunnel: w456 -> [_ w475]
                    frame #0 {
                      n176 = local write "error?"(w466) -> ()
                    }
                    frame #1 {
                      n177 = local read "Mode 4"() -> (w473:u16)
                      n178 = call "compliancevi3subvi.vi"("compliance (A)"=w467, "start"=w469, "compliance (V)"=w468, "total points"=w474, "step"=w471, "Mode"=w473) -> ("total points 2"=w470:u16, "compliance"=w472:dbl)  [unwired: 1 in, 1 out]
                      n179 = call "HP415xA _Config-Sweep-Secondary Sour.vi"("compliance"=w472, "step"=w471, "error in (no error)"=w477, "total points"=w470, "start"=w469, "VISA session"=w475) -> ("error out"=w476:errorcluster)  [unwired: 1 in]
                      n180 = local write "error?"(w476) -> ()
                    }
                  }
                }
                frame #1 {
                  n181 = local read "Mode 3"() -> (w488:u16)
                  n182 = call "compliancevi3subvi.vi"("compliance (A)"=w479, "start"=w481, "compliance (V)"=w478, "total points"=w484, "step"=w480, "Mode"=w488) -> ("total points 2"=w483:u16, "compliance"=w482:dbl)  [unwired: 1 in, 1 out]
                  n183 = call "HP415xA _Config-Sweep-Secondary Sour.vi"("compliance"=w482, "step"=w480, "error in (no error)"=w487, "total points"=w483, "start"=w481, "VISA session"=w485) -> ("error out"=w486:errorcluster)  [unwired: 1 in]
                  n184 = local write "error?"(w486) -> ()
                }
              }
            }
            frame #1 {
              n185 = local read "Mode 2"() -> (w499:u16)
              n186 = call "compliancevi3subvi.vi"("compliance (A)"=w495, "start"=w491, "compliance (V)"=w494, "total points"=w493, "step"=w489, "Mode"=w499) -> ("total points 2"=w492:u16, "compliance"=w490:dbl)  [unwired: 1 in, 1 out]
              n187 = call "HP415xA _Config-Sweep-Secondary Sour.vi"("compliance"=w490, "step"=w489, "error in (no error)"=w498, "total points"=w492, "start"=w491, "VISA session"=w496) -> ("error out"=w497:errorcluster)  [unwired: 1 in]
              n188 = local write "error?"(w497) -> ()
            }
          }
        }
      }
    }
    frame #4 {
      # "This step sets the integration time."
      n189 = local read "VISA session"() -> (w500:refnum<visa-resource-name>)
      n190 = local read "error?"() -> (w504:errorcluster)
      n191 = call "HP415xA _Config-Meas-Timing.vi"("error in (no error)"=w504, "wait time parameter"="wait time parameter", "integration time"="integration time", "VISA session"=w500) -> ("error out"=w503:errorcluster)  [unwired: 2 in]
      n192 = local write "error?"(w503) -> ()
    }
    frame #5 {
      w532 = u32 1 items=["stop  ", "single  ", "single-append  ", "stress start  ", "continuous  ", "standby on  ", "standby off  ", "zero  "] ("function (stop:0)")
      w536 = u16 2 items=["disabled", "Var1", "Var2", "Var1'", "Constant"] ("Function")
      w541 = u16 1 items=["disabled", "Var1", "Var2", "Var1'", "Constant"] ("Function")
      n193 = local read "Function"() -> (w543:u16)
      n194 = local read "Function"() -> (w535:u16)
      n195 = Equal?(x=w543, y=w541) -> (x = y?=w542:bool)
      n196 = Equal?(x=w535, y=w536) -> (x = y?=w534:bool)
      n197 = case shown="False" w542 {
        tunnel: [w737 w752] -> w537
        tunnel: [w738 w751] -> _
        tunnel: w541 -> [w735 _]
        frame #0 {
          n198 = local read "Function 2"() -> (w739:u16)
          n199 = Equal?(x=w739, y=w735) -> (x = y?=w736:bool)
          n200 = case shown="False" w736 {
            tunnel: [w740 w750] -> w738
            tunnel: [w741 w749] -> w737
            tunnel: w735 -> [w744 _]
            frame #0 {
              n201 = local read "Function 3"() -> (w743:u16)
              n202 = Equal?(x=w743, y=w744) -> (x = y?=w742:bool)
              n203 = case shown="True" w742 {
                tunnel: [w746 w748] -> w741
                tunnel: [w745 w747] -> w740
                frame #0 {
                  n204 = local read "Vname 4"() -> (w746:string)
                  n205 = local read "Iname 4"() -> (w745:string)
                }
                frame #1 {
                  n206 = local read "Vname 3"() -> (w748:string)
                  n207 = local read "Iname 3"() -> (w747:string)
                }
              }
            }
            frame #1 {
              n208 = local read "Vname 2"() -> (w749:string)
              n209 = local read "Iname 2"() -> (w750:string)
            }
          }
        }
        frame #1 {
          n210 = local read "Vname"() -> (w752:string)
          n211 = local read "Iname"() -> (w751:string)
        }
      }
      n212 = case shown="False" w534 {
        tunnel: [w627 w680] -> w507
        tunnel: [w626 TRUE ("x = y?")] -> w512
        frame #0 {
          w630 = u16 2 items=["disabled", "Var1", "Var2", "Var1'", "Constant"] ("Function")
          n213 = local read "Function 2"() -> (w629:u16)
          n214 = Equal?(x=w629, y=w630) -> (x = y?=w628:bool)
          n215 = case shown="True" w628 {
            tunnel: [w632 w670] -> w627
            tunnel: [w631 TRUE ("x = y?")] -> w626
            frame #0 {
              w635 = u16 2 items=["disabled", "Var1", "Var2", "Var1'", "Constant"] ("Function")
              n216 = local read "Function 3"() -> (w634:u16)
              n217 = Equal?(x=w634, y=w635) -> (x = y?=w633:bool)
              n218 = case shown="False" w633 {
                tunnel: [w640 w660] -> w632
                tunnel: [w636 TRUE ("x = y?")] -> w631
                frame #0 {
                  w639 = u16 2 items=["disabled", "Var1", "Var2", "Var1'", "Constant"] ("Function")
                  n219 = local read "Function 4"() -> (w638:u16)
                  n220 = Equal?(x=w638, y=w639) -> (x = y?=w637:bool)
                  n221 = case shown="True" w637 {
                    tunnel: ["0" ("Vname 4") w650] -> w640
                    tunnel: [FALSE ("x = y?") TRUE ("x = y?")] -> w636
                    frame #0 {
                    }
                    frame #1 {
                      w644 = u16 2 items=["V", "I", "VPulse", "IPulse", "Common"] ("Mode 2")
                      w647 = u16 0 items=["V", "I", "VPulse", "IPulse", "Common"] ("Mode 2")
                      n222 = local read "Mode 4"() -> (w646:u16)
                      n223 = Equal?(x=w647, y=w646) -> (x = y?=w648:bool)
                      n224 = Equal?(x=w646, y=w644) -> (x = y?=w645:bool)
                      n225 = Or(x=w648, y=w645) -> (x .or. y?=w643:bool)
                      n226 = case shown="False" w643 {
                        tunnel: [w651 w652] -> w650
                        frame #0 {
                          n227 = local read "Iname 4"() -> (w651:string)
                        }
                        frame #1 {
                          n228 = local read "Vname 4"() -> (w652:string)
                        }
                      }
                    }
                  }
                }
                frame #1 {
                  w656 = u16 2 items=["V", "I", "VPulse", "IPulse", "Common"] ("Mode 2")
                  w655 = u16 0 items=["V", "I", "VPulse", "IPulse", "Common"] ("Mode 2")
                  n229 = local read "Mode 3"() -> (w654:u16)
                  n230 = Equal?(x=w655, y=w654) -> (x = y?=w658:bool)
                  n231 = Equal?(x=w654, y=w656) -> (x = y?=w657:bool)
                  n232 = Or(x=w658, y=w657) -> (x .or. y?=w653:bool)
                  n233 = case shown="False" w653 {
                    tunnel: [w661 w662] -> w660
                    frame #0 {
                      n234 = local read "Iname 3"() -> (w661:string)
                    }
                    frame #1 {
                      n235 = local read "Vname 3"() -> (w662:string)
                    }
                  }
                }
              }
            }
            frame #1 {
              w664 = u16 2 items=["V", "I", "VPulse", "IPulse", "Common"] ("Mode 2")
              w665 = u16 0 items=["V", "I", "VPulse", "IPulse", "Common"] ("Mode 2")
              n236 = local read "Mode 2"() -> (w666:u16)
              n237 = Equal?(x=w665, y=w666) -> (x = y?=w668:bool)
              n238 = Equal?(x=w666, y=w664) -> (x = y?=w667:bool)
              n239 = Or(x=w668, y=w667) -> (x .or. y?=w663:bool)
              n240 = case shown="True" w663 {
                tunnel: [w671 w672] -> w670
                frame #0 {
                  n241 = local read "Iname 2"() -> (w671:string)
                }
                frame #1 {
                  n242 = local read "Vname 2"() -> (w672:string)
                }
              }
            }
          }
        }
        frame #1 {
          w677 = u16 2 items=["V", "I", "VPulse", "IPulse", "Common"] ("Mode")
          w678 = u16 0 items=["V", "I", "VPulse", "IPulse", "Common"] ("Mode")
          n243 = local read "Mode"() -> (w676:u16)
          n244 = Equal?(x=w676, y=w678) -> (x = y?=w675:bool)
          n245 = Equal?(x=w676, y=w677) -> (x = y?=w674:bool)
          n246 = Or(x=w675, y=w674) -> (x .or. y?=w673:bool)
          n247 = case shown="True" w673 {
            tunnel: [w681 w682] -> w680
            frame #0 {
              n248 = local read "Iname"() -> (w681:string)
            }
            frame #1 {
              n249 = local read "Vname"() -> (w682:string)
            }
          }
        }
      }
      n250 = local read "error?"() -> (w524:errorcluster)
      n251 = Unbundle("Y2 axis settings") -> ("Y2 axis on/off"=w514:bool, "MINIMUM"=w529:ext, "MAXIMUM"=w528:ext, "Variable name"=w521:string, "LIN or LOG axis"=w527:string)
      n252 = local read "Var2 step settings"() -> (w539:T2)
      n253 = local read "Var1 sweep settings"() -> (w540:T3)
      n254 = Unbundle(w539) -> ("total points"=w538:u16)  [unwired: 4 out]
      n255 = local read "VISA session"() -> (w519:refnum<visa-resource-name>)
      n256 = call "Y1subvi.vi"("MAXIMUM"="MAXIMUM", "Variable name"="Y1 axis", "error in (no error)"=w524, "MINIMUM"="MINIMUM", "LIN or LOG axis"="LIN", "VISA resource name"=w519) -> ("error out"=w525:errorcluster)
      n257 = case shown="True" w514 {
        tunnel: w525 -> [w618 w625]
        tunnel: w519 -> [_ w624]
        tunnel: w529 -> [_ w623]
        tunnel: w528 -> [_ w622]
        tunnel: w521 -> [_ w621]
        tunnel: w527 -> [_ w620]
        tunnel: [w618 w619] -> w526
        frame #0 {
        }
        frame #1 {
          n258 = call "Y2subvi.vi"("MAXIMUM"=w622, "Variable name"=w621, "error in (no error)"=w625, "MINIMUM"=w623, "LIN or LOG axis"=w620, "VISA resource name"=w624) -> ("error out"=w619:errorcluster)
        }
      }
      n259 = Decrement(x=w538) -> (x-1=w513:u16)
      n260 = Unbundle(w540) -> ("start"=w510:dbl)  [unwired: 6 out]
      n261 = call "HP415xA Op-Start-Stop.vi"("error in (no error)"=w526, "function (stop:0)"=w532, "wait until finish"=TRUE, "VISA session"=w519) -> ("error out"=w531:errorcluster)  [unwired: 6 in, 1 out]
      n262 = call "HP415xA Op-Download Trace.vi"("error in (no error)"=w531, "trace (variable) name"=w537, "VISA session"=w519) -> ("error out"=w546:errorcluster, "trace"=w511:dbl[])
      n263 = call "HP415xA Op-Download Trace.vi"("error in (no error)"=w546, "trace (variable) name"="Y1 axis", "VISA session"=w519) -> ("error out"=w522:errorcluster, "trace"=w516:dbl[])
      n264 = case shown="True" w514 {
        tunnel: w522 -> [w603 w611]
        tunnel: w519 -> [_ w610]
        tunnel: w521 -> [_ w609]
        tunnel: [w603 w608] -> w520
        tunnel: w511 -> [w601 w607]
        tunnel: w516 -> [w602 w606]
        tunnel: [w600 w605] -> w515
        tunnel: [dbl[] [] ("trace") w604] -> w509
        frame #0 {
          n265 = Bundle("trace"=w601, "trace"=w602) -> (w600:cluster{"trace":dbl[], "trace":dbl[]})  [unwired: 1 in]
        }
        frame #1 {
          n266 = call "HP415xA Op-Download Trace.vi"("error in (no error)"=w611, "trace (variable) name"=w609, "VISA session"=w610) -> ("error out"=w608:errorcluster, "trace"=w604:dbl[])
          n267 = stacked-sequence {
            tunnel: w604 -> [_ w616]
            tunnel: w607 -> [w614 w615]
            tunnel: w606 -> [w613 _]
            tunnel: [w612 _] -> w605
            frame #0 {
              n268 = Bundle("trace"=w614, "trace"=w613) -> (w612:cluster{"trace":dbl[], "trace":dbl[]})  [unwired: 1 in]
            }
            frame #1 {
              n269 = Bundle("trace"=w615, "trace"=w616) -> (→"graphic display 2":cluster{"trace":dbl[], "trace":dbl[]})  [unwired: 1 in]
            }
          }
        }
      }
      "graphic display" <- w515
      n270 = case shown="True" w512 {
        tunnel: w510 -> [_ w720]
        tunnel: w516 -> [w687 w719]
        tunnel: w511 -> [w688 w717]
        tunnel: w513 -> [_ w710]
        tunnel: w513 -> [_ w699]
        tunnel: w519 -> [_ w698]
        tunnel: w520 -> [_ w697]
        tunnel: [w689 w696] -> w506
        tunnel: w507 -> [_ w695]
        tunnel: w507 -> [_ w693]
        tunnel: [dbl[] [] ("trace") w690] -> w508
        frame #0 {
          n271 = Build Array(w688, w687) -> (w684:dbl[][])
          n272 = local read "error?"() -> (w689:errorcluster)
          n273 = call-poly <vilib>:"Write To Spreadsheet File.vi"("transpose? (no:F)"=TRUE ("append to file? (new file:F)"), "format (%.3f)"="%.5e", "2D data"=w684) -> ()  [unwired: 5 in, 1 out]
        }
        frame #1 {
          n274 = call "HP415xA Op-Download Trace.vi"("error in (no error)"=w697, "trace (variable) name"=w695, "VISA session"=w698) -> ("error out"=w696:errorcluster, "trace"=w690:dbl[])
          n275 = for {
            N: w710 -> [_]
            shift-right: [w731] -> w716
            shift-left: w717 -> [w727]
            tunnel: w720 -> [w733]
            tunnel: [w732] -> _ mode=indexing
            shift-right: [w728] -> w715
            shift-left: w719 -> [w730]
            tunnel: [w729] -> w718 mode=indexing
            shift-right: [w722] -> w713
            shift-left: w690 -> [w726]
            tunnel: [w724] -> w714 mode=indexing
            n276 = Search 1D Array(1D array=w727, element=w733, start index (0)=1) -> (index of element=w723:i32)
            n277 = Split 1D Array(array=w726, index=w723) -> (first subarray=w721:dbl[], second subarray=w722:dbl[])
            n278 = Split 1D Array(array=w730, index=w723) -> (first subarray=w729:dbl[], second subarray=w728:dbl[])
            n279 = Split 1D Array(array=w727, index=w723) -> (first subarray=w732:dbl[], second subarray=w731:dbl[])
            n280 = Index Array(array=w721, index=1) -> (element=w724:dbl)
          }
          n281 = Index Array(array=w713, index=1) -> (element=w711:dbl)
          n282 = Insert Into Array(array=w714, index=w699, new element=w711) -> (w705:dbl[])
          n283 = Build Array (concatenate)(w716, w718, w715) -> (w709:dbl[][])
          n284 = Array To Spreadsheet String(delimiter (Tab)=",", array=w705, 3:"%.5e" ("format string")) -> (spreadsheet string=w694:string)
          n285 = Concatenate Strings(w693, "," ("string")) -> (w691:string)
          n286 = Transpose 2D Array(2D array=w709) -> (transposed array=w703:dbl[][])
          n287 = Concatenate Strings(w691, w694) -> (w702:string)
          n288 = Array To Spreadsheet String(delimiter (Tab)=",", array=w703, 3:"%.5e" ("format string")) -> (spreadsheet string=w701:string)
          n289 = Concatenate Strings(w702, w701) -> (w700:string)
          n290 = call <vilib>:"Write Characters To File.vi"("character string"=w700) -> ()  [unwired: 4 in, 1 out]
        }
      }
      n291 = case shown="True" w514 {
        tunnel: w513 -> [_ w552]
        tunnel: w512 -> [_ w553]
        tunnel: w511 -> [_ w551]
        tunnel: w510 -> [_ w550]
        tunnel: w509 -> [_ w549]
        tunnel: w508 -> [_ w548]
        tunnel: w507 -> [_ w547]
        frame #0 {
        }
        frame #1 {
          n292 = case shown="True" w553 {
            tunnel: w552 -> [_ w569]
            tunnel: w551 -> [w557 w584]
            tunnel: w550 -> [_ w583]
            tunnel: w549 -> [w558 w582]
            tunnel: w548 -> [_ w581]
            tunnel: w547 -> [_ w564]
            frame #0 {
              n293 = Build Array(w557, w558) -> (w556:dbl[][])
              n294 = call-poly <vilib>:"Write To Spreadsheet File.vi"("transpose? (no:F)"=TRUE, "format (%.3f)"="%.5e", "2D data"=w556) -> ()  [unwired: 5 in, 1 out]
            }
            frame #1 {
              n295 = for {
                N: w569 -> [_]
                shift-right: [w595] -> w580
                shift-left: w584 -> [w596]
                tunnel: w583 -> [w598]
                tunnel: [w594] -> _ mode=indexing
                shift-right: [w591] -> w578
                shift-left: w582 -> [w593]
                tunnel: [w592] -> w579 mode=indexing
                shift-right: [w588] -> w573
                shift-left: w581 -> [w589]
                tunnel: [w585] -> w570 mode=indexing
                n296 = Search 1D Array(1D array=w596, element=w598, start index (0)=1) -> (index of element=w590:i32)
                n297 = Split 1D Array(array=w596, index=w590) -> (first subarray=w594:dbl[], second subarray=w595:dbl[])
                n298 = Split 1D Array(array=w593, index=w590) -> (first subarray=w592:dbl[], second subarray=w591:dbl[])
                n299 = Split 1D Array(array=w589, index=w590) -> (first subarray=w586:dbl[], second subarray=w588:dbl[])
                n300 = Index Array(array=w586, index=1) -> (element=w585:dbl)
              }
              n301 = Build Array (concatenate)(w580, w579, w578) -> (w577:dbl[][])
              n302 = Index Array(array=w573, index=1) -> (element=w571:dbl)
              n303 = Transpose 2D Array(2D array=w577) -> (transposed array=w576:dbl[][])
              n304 = Insert Into Array(array=w570, index=w569, new element=w571) -> (w568:dbl[])
              n305 = Array To Spreadsheet String(delimiter (Tab)=",", array=w568, 3:"%.5e" ("format string")) -> (spreadsheet string=w562:string)
              n306 = Array To Spreadsheet String(delimiter (Tab)=",", array=w576, 3:"%.5e" ("format string")) -> (spreadsheet string=w560:string)
              n307 = Concatenate Strings(w564, "," ("string")) -> (w563:string)
              n308 = Concatenate Strings(w563, w562) -> (w561:string)
              n309 = Concatenate Strings(w561, w560) -> (w559:string)
              n310 = call <vilib>:"Write Characters To File.vi"("character string"=w559) -> ()  [unwired: 4 in, 1 out]
            }
          }
        }
      }
      n311 = call "HP415xA Sys-Error Query.vi"("VISA session"=w519, "error in (no error)"=w506) -> ("error out"=w544:errorcluster)  [unwired: 2 in, 1 out]
      n312 = call "HP415xA  Close.vi"("error in (no error)"=w544, "VISA session"=w519) -> ("error out"=w545:errorcluster)
      n313 = local write "error?"(w545) -> ()
    }
  }
